vi "Configure Trigger Modifier.vi"(8 "error in (no error)":errorcluster, 9 "Trigger Type":u16(ring) items=["Edge", "Pulse", "TV", "Pattern"], 10 "Trigger Modifier (0: Auto)":u16(ring) items=["Auto", "Normal", "Single"], 11 "VISA resource name":refnum<visa-resource-name>) -> (0 "error out":errorcluster, 3 "VISA resource name out":refnum<visa-resource-name>)   [LabVIEW 2010, in "Agilent DSO1000 Series.lvlib"]
doc: "This VI configures trigger sweep mode."
uses:
  <instrlib>/Agilent DSO1000 Series/Agilent DSO1000 Series.lvlib
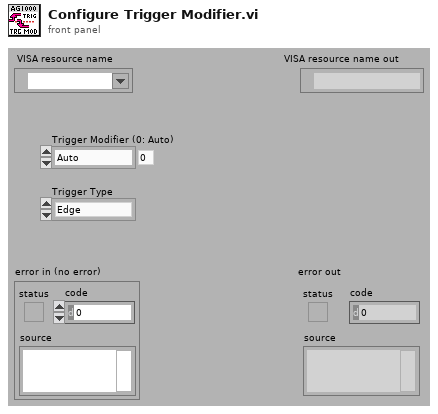
[diagram p1: front panel]
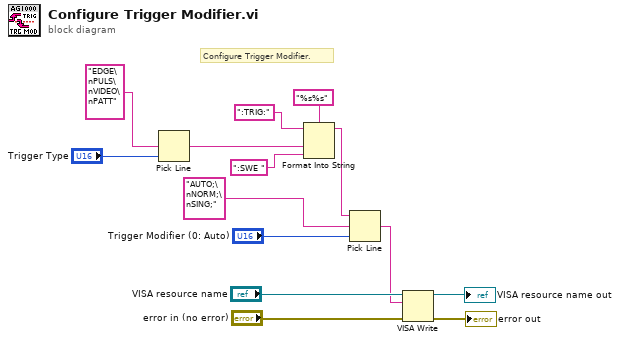
[diagram p0: block diagram]
diagram:
  # "Configure Trigger Modifier."
  n1 = Pick Line(multi-line string="EDGE\nPULS\nVIDEO\nPATT", line index="Trigger Type") -> (output string=w7:string)  [unwired: 1 in]
  n2 = Format Into String(format string="%s%s", initial string=":TRIG:", w7, ":SWE ") -> (resulting string=w4:string)  [unwired: 1 in, 1 out]
  n3 = Pick Line(string ("")=w4, multi-line string="AUTO;\nNORM;\nSING;", line index="Trigger Modifier (0: Auto)") -> (output string=w10:string)
  n4 = VISA Write(VISA resource name="VISA resource name", write buffer=w10, error in (no error)="error in (no error)") -> (VISA resource name out=→"VISA resource name out":refnum<visa-resource-name>, error out=→"error out":errorcluster)  [unwired: 1 out]
